vi "practica8.vi"() -> ()   [LabVIEW 2016]
panel:
  out "Waveform Graph":dbl[](graph)
  out "second subarray":dbl[](array[numeric])
  out "number":dbl[](array[numeric])
  out "text":string[](array[string])
  in  "file path (use dialog)":path
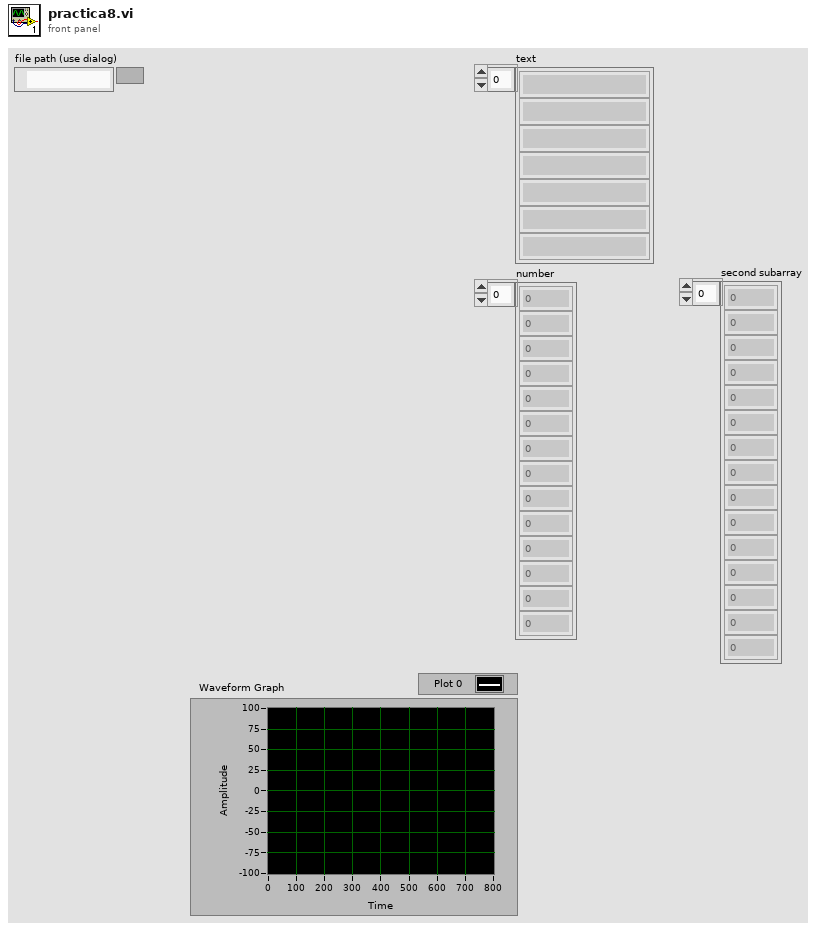
[diagram p1: front panel]
types:
  T1 = enum16{"open", "replace", "create", "open or create", "replace or create", "replace or create with confirmation"}
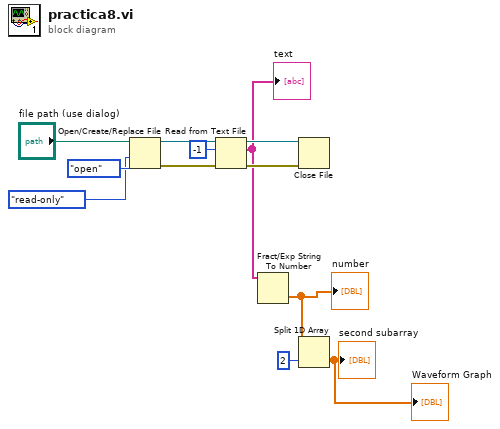
[diagram p0: block diagram]
diagram:
  n1 = Open/Create/Replace File(file path (use dialog)="file path (use dialog)", operation (0:open)=T1."open", access (0:read/write)=enum16{"read/write", "read-only", "write-only"}."read-only") -> (refnum out=w10:refnum<file>, error out=w8:errorcluster)  [unwired: 3 in, 1 out]
  n2 = Read from Text File(file (use dialog)=w10, count=-1, error in=w8) -> (refnum out=w11:refnum<file>, text=w4:string[], error out=w9:errorcluster)  [unwired: 1 in, 1 out]
  "text" <- w4
  n3 = Fract/Exp String To Number(string=w4) -> (number=w3:dbl[])  [unwired: 3 in, 1 out]
  "number" <- w3
  n4 = Close File(refnum=w11, error in=w9) -> ()  [unwired: 2 out]
  n5 = Split 1D Array(array=w3, index=2) -> (second subarray=→"second subarray" →"Waveform Graph":dbl[])  [unwired: 1 out]
